vi "XYZtoRGB.vi"(1 "XYZ":dbl[](array[numeric]), 2 "Illuminants":T1, 3 "Selected RGB":string(combo)) -> (0 "RGB":dbl[](array[numeric]))   [LabVIEW 2013]
uses:
  <vilib>/Analysis/baseanly.llb/A x Vector.vi
  <vilib>/Analysis/baseanly.llb/Real Inverse Matrix.vi
  <vilib>/Analysis/NI_AALBase.lvlib
panel:
  out "XYZd":dbl[](array[numeric])
  out "RGB sem gama":dbl[](array[numeric]) format="%#.7f"
  out "gamma":dbl
  out "RGBMatrix":dbl[][](array[numeric])
  out "M^-1":dbl[][](array[numeric])
  out "RGBStandardRows":i32
  out "RGBStandards":string[][](array[string])
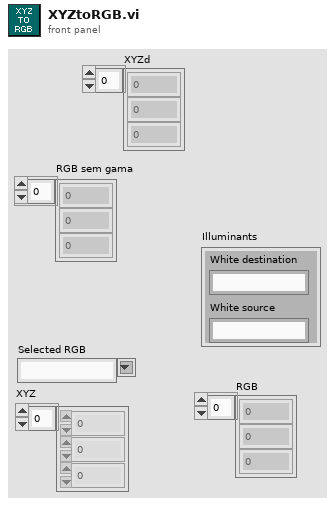
[diagram p1: front panel]
types:
  T1 = cluster{"White destination":string, "White source":string}
  T2 = typedef "NI_Matrix.lvlib/RealMatrix.ctl" = dbl[][]
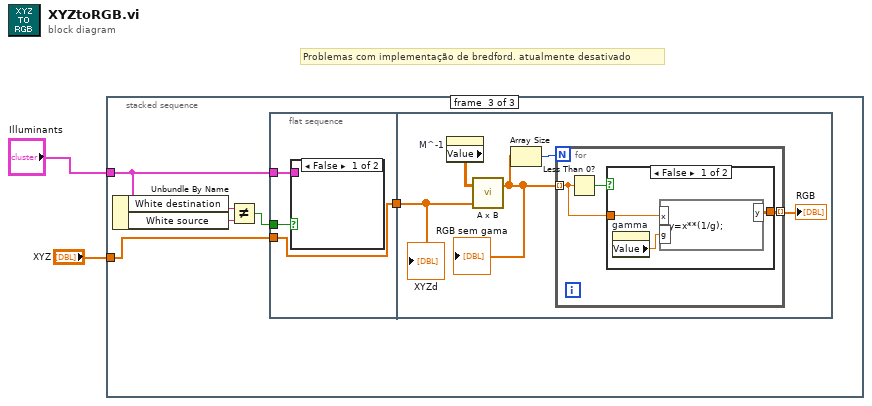
[diagram p0: block diagram]
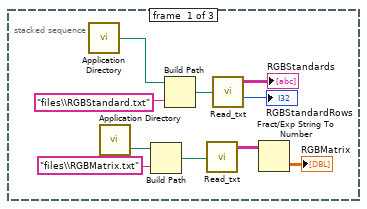
[diagram p2: hidden frame]
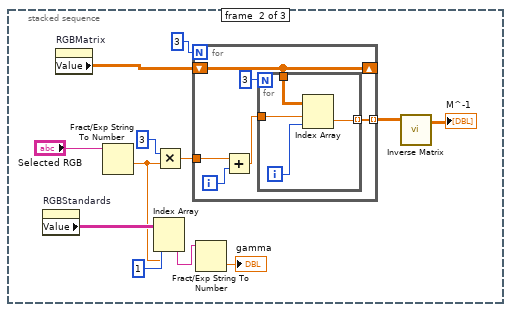
[diagram p3: hidden frame]
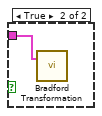
[diagram p4: hidden frame]
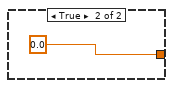
[diagram p5: hidden frame]
diagram:
  # "Problemas com implementação de bredford. atualmente desativado"
  n1 = stacked-sequence {
    tunnel: "XYZ" -> [_ _ w40]
    tunnel: "Illuminants" -> [_ _ w39]
    frame #0 {
      n2 = call <vilib>:"Application Directory.vi"() -> ("Application Directory"=w4:path)
      n3 = call <vilib>:"Application Directory.vi"() -> ("Application Directory"=w3:path)
      n4 = Build Path(base path=w3, name or relative path="files\\RGBMatrix.txt") -> (appended path=w7:path)
      n5 = Build Path(base path=w4, name or relative path="files\\RGBStandard.txt") -> (appended path=w5:path)
      n6 = call "Read_txt.vi"("file path (dialog if empty)"=w7) -> ("Elements"=w9:string[][])  [unwired: 2 out]
      n7 = call "Read_txt.vi"("file path (dialog if empty)"=w5) -> ("Elements"=→"RGBStandards":string[][], "Rows"=→"RGBStandardRows":i32)  [unwired: 1 out]
      n8 = Fract/Exp String To Number(string=w9) -> (number=→"RGBMatrix":dbl[][])  [unwired: 3 in, 1 out]
    }
    frame #1 {
      n9 = property on="RGBStandards" class="Arr (strict)"() -> ("Value"=w17:string[][])  [unwired: 2 in, 2 out]
      n10 = property on="RGBMatrix" class="Arr (strict)"() -> ("Value"=w21:dbl[][])  [unwired: 2 in, 2 out]
      n11 = Fract/Exp String To Number(string="Selected RGB") -> (number=w15:dbl)  [unwired: 3 in, 1 out]
      n12 = Index Array(array=w17, index (row)=w15, index (col)=1 ("disabled index (col)")) -> (element=w14:string)
      n13 = Multiply(x=3, y=w15) -> (x*y=w22:dbl)
      n14 = for {
        N: 3 -> [_]
        shift-right: [w29] -> _
        shift-left: w21 -> [w29]
        tunnel: w22 -> [w28]
        tunnel: [w25] -> w19 mode=indexing
        i -> [w27]
        n15 = Add(x=w28, y=w27) -> (x+y=w26:dbl)
        n16 = for {
          N: 3 -> [_]
          tunnel: w29 -> [w34]
          tunnel: w26 -> [w33]
          tunnel: [w32] -> w25 mode=indexing
          i -> [w31]
          n17 = Index Array(array=w34, index (row)=w33, index (col)=w31) -> (element=w32:dbl)
        }
      }
      n18 = Fract/Exp String To Number(string=w14) -> (number=→"gamma":dbl)  [unwired: 3 in, 1 out]
      n19 = call-poly <vilib>:"Inverse Matrix.vi"("Input Matrix"=w19) -> ("Inverse Matrix"=→"M^-1":T2)  [unwired: 1 in, 1 out]
    }
    frame #2 {
      n20 = Unbundle By Name(w39) -> ("White destination"=w37:string, "White source"=w38:string)
      n21 = Not Equal?(x=w37, y=w38) -> (x != y?=w36:bool)
      n22 = flat-sequence {
        tunnel: w36 -> [w43]
        tunnel: w40 -> [w41]
        tunnel: w39 -> [w42]
        tunnel: [w41] -> w35
        tunnel: w35 -> [w46]
        frame #0 {
          n23 = case shown="False" w43 {
            tunnel: w42 -> [_ w44]
            frame False {
            }
            frame True {
              n24 = call "Bradford Transformation.vi"("Illuminants"=w44) -> ()  [unwired: 1 in, 1 out]
            }
          }
        }
        frame #1 {
          n25 = property on="M^-1" class="Arr (strict)"() -> ("Value"=w47:dbl[][])  [unwired: 2 in, 2 out]
          n26 = call-poly <vilib>:"A x B.vi"("Vector"=w46, "A"=w47) -> ("A x Vector"=w49:dbl[])  [unwired: 1 out]
          "RGB sem gama" <- w49
          n27 = Array Size(array=w49) -> (size(s)=w45:i32)
          n28 = for {
            N: w45 -> [_]
            tunnel: w49 -> [w51] mode=indexing
            tunnel: [w52] -> w48 mode=indexing
            n29 = Less Than 0?(x=w51) -> (x < 0?=w50:bool)
            n30 = case shown="False" w50 {
              tunnel: [w54 0.0] -> w52
              tunnel: w51 -> [w55 _]
              frame False {
                n31 = property on="gamma" class="DigNum (strict)"() -> ("Value"=w53:dbl)  [unwired: 2 in, 2 out]
                n32 = formula code="y=x**(1/g);"("x"=w55, "g"=w53) -> ("y"=w54:dbl)
              }
              frame True {
              }
            }
          }
          "RGB" <- w48
          "XYZd" <- w46
        }
      }
    }
  }
